vi "ProgG_005_kz_podprogram.vi"(10 "x2":ext=19.4, 11 "x1":ext=14.1) -> (3 "Numeric":ext=14.1049999999999999996)   [LabVIEW 2021]
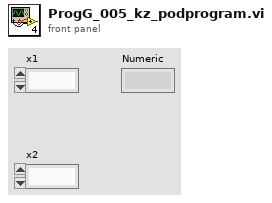
[diagram p1: front panel]
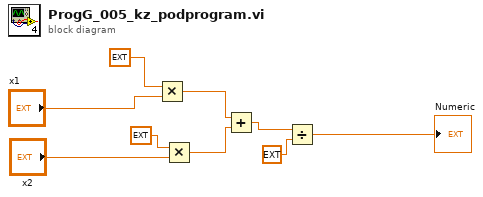
[diagram p0: block diagram]
diagram:
  n1 = Multiply(x=ext 0.9, y="x1") -> (x*y=w5:ext)
  n2 = Multiply(x=ext 0.8, y="x2") -> (x*y=w6:ext)
  n3 = Add(x=w5, y=w6) -> (x+y=w7:ext)
  n4 = Divide(x=w7, y=ext 2.0) -> (x/y=→"Numeric":ext)
